vi "UTIL_RegEdit.vi"(9 "Mode":enum16{"Write", "Read", "Delete"}(ring), 10 "String Name":string="My String", 11 "String Value":string="LabVIEW") -> (2 "Success?":bool, 3 "Value Read":string)   [LabVIEW 2024]
doc: "This example demonstrates how to write, read, and delete a sample key from the Windows registry key HKEY_CURRENT_USER\\Allen_Aircraft\\. It will not affect the registry in any other way."
uses:
  <vilib>/registry/registry.llb/Registry RtKey.ctl
  <vilib>/registry/registry.llb/Write Registry Value Simple.vi
  <vilib>/registry/registry.llb/Read Registry Value Simple STR.vi
panel:
  # "Overview: Demonstrates the use of the Windows Registry Access VIs to write, read, and delete a sample key from the Windows registry.\nRequirements: Windows\nInstructions:\nRun the VI."
  # "KEY PATH:  HKEY_CURRENT_USER\\Allen_Aircraft\\Elevale_OLS_Test"
  # "See the diagram of this VI for more information on the Windows Registry Access VIs."
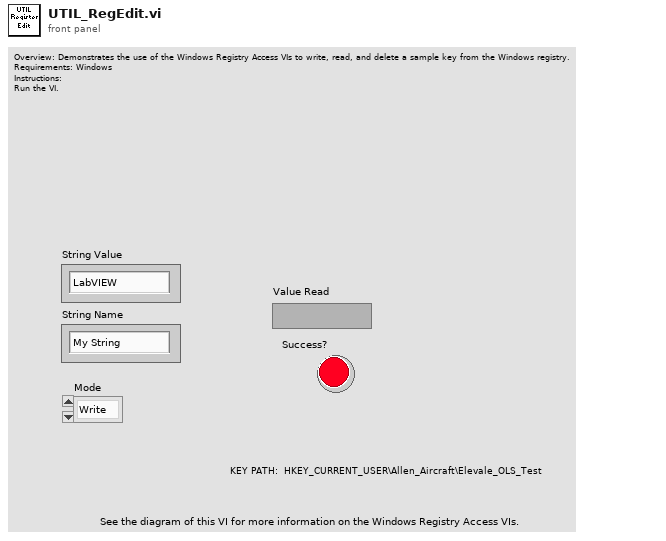
[diagram p1: front panel]
types:
  T1 = typedef "Registry RtKey.ctl" = enum32{"HKEY_CLASSES_ROOT", "HKEY_CURRENT_USER", "HKEY_LOCAL_MACHINE", "HKEY_USERS", "HKEY_PERFORMANCE_DATA", "HKEY_CURRENT_CONFIG", "HKEY_DYN_DATA"}
  T2 = typedef "Registry refnum.ctl" = refnum<k1>
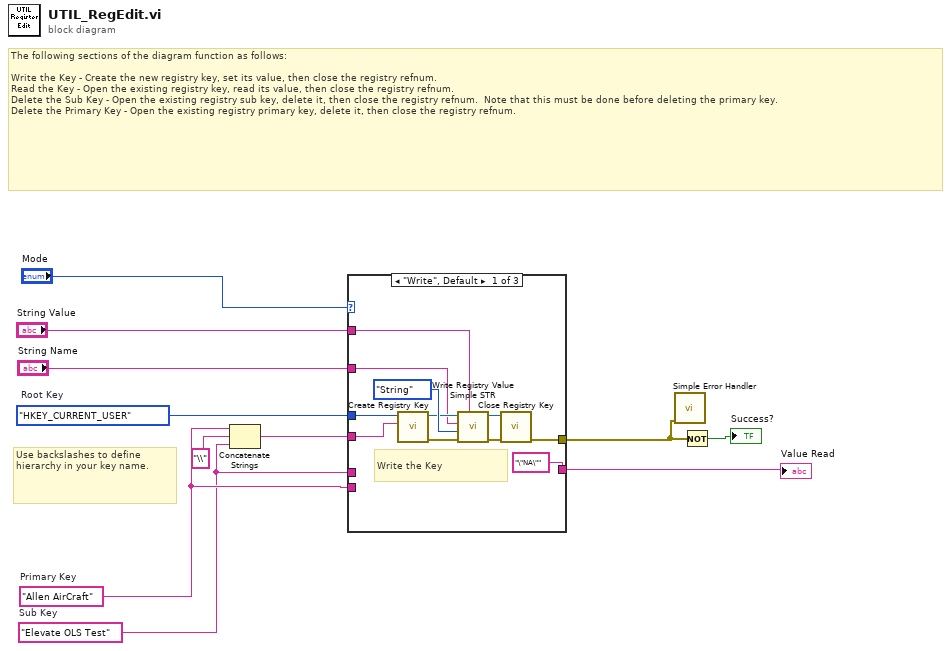
[diagram p0: block diagram]
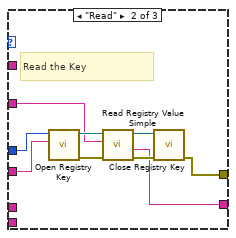
[diagram p2: hidden frame]
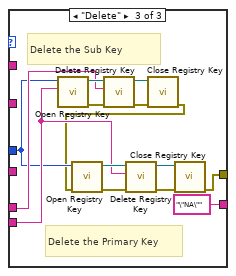
[diagram p3: hidden frame]
diagram:
  w2 = "Elevate OLS Test"  # Sub Key
  w3 = "Allen AirCraft"  # Primary Key
  w11 = Registry_RtKey."HKEY_CURRENT_USER"  # Root Key
  # "Use backslashes to define hierarchy in your key name."
  # "The following sections of the diagram function as follows:\n\nWrite the Key - Create the new registry key, set its value, then close the registry refnum.\nRead the Key - Open the existing registry key, read its value, then close the registry refnum.\nDelete the Sub Key - Open the existing registry sub key, delete it, then close the registry refnum.  Note that this must be done before deleting the primary key.\nDelete the Primary Key - Open the existing registry primary key, delete it, then close the registry refnum."
  n1 = Concatenate Strings(w3, "\\", w2) -> (w10:string)
  n2 = case shown="\"Write\", Default" "Mode" {
    tunnel: w11 -> [w17 w25 w35]
    tunnel: w10 -> [w16 w24 _]
    tunnel: [w15 w27 w33] -> w1
    tunnel: "String Name" -> [w14 w26 _]
    tunnel: "String Value" -> [w13 _ _]
    tunnel: ["\"NA\"" ("String/Binary data") w23 "\"NA\"" ("String/Binary data")] -> w4
    tunnel: w3 -> [_ _ w36]
    tunnel: w2 -> [_ _ w41]
    frame "Write", Default {
      # "Write the Key"
      n3 = call <vilib>:"Create Registry Key.vi"("subkey"=w16, "root key (HKEY_LOCAL_MACHINE)"=w17) -> ("error out"=w20:errorcluster, "refnum out"=w18:T2)  [unwired: 7 in, 1 out]
      n4 = call-poly <vilib>:"Write Registry Value Simple STR.vi"("String/Binary data"=w13, "error in (no error)"=w20, "simple data type"=enum16{"String", "Binary", "DWORD"}."String", "value"=w14, "refnum"=w18) -> ("error out"=w22:errorcluster, "refnum out"=w21:T2)  [unwired: 3 in]
      n5 = call <vilib>:"Close Registry Key.vi"("error in (no error)"=w22, "refnum"=w21) -> ("error out"=w15:errorcluster)  [unwired: 5 in]
    }
    frame "Read" {
      # "Read the Key"
      n6 = call <vilib>:"Open Registry Key.vi"("subkey"=w24, "root key (HKEY_LOCAL_MACHINE)"=w25) -> ("error out"=w31:errorcluster, "refnum out"=w30:T2)  [unwired: 8 in]
      n7 = call-poly <vilib>:"Read Registry Value Simple.vi"("error in (no error)"=w31, "value"=w26, "refnum"=w30) -> ("error out"=w28:errorcluster, "String/Binary data"=w23:string, "refnum out"=w29:T2)  [unwired: 3 in, 1 out]
      n8 = call <vilib>:"Close Registry Key.vi"("error in (no error)"=w28, "refnum"=w29) -> ("error out"=w27:errorcluster)  [unwired: 5 in]
    }
    frame "Delete" {
      # "Delete the Primary Key"
      # "Delete the Sub Key"
      n9 = call <vilib>:"Open Registry Key.vi"("subkey"=w36, "root key (HKEY_LOCAL_MACHINE)"=w35) -> ("error out"=w42:errorcluster, "refnum out"=w43:T2)  [unwired: 8 in]
      n10 = call <vilib>:"Delete Registry Key.vi"("error in (no error)"=w42, "subkey"=w41, "refnum"=w43) -> ("error out"=w44:errorcluster, "refnum out"=w45:T2)  [unwired: 7 in]
      n11 = call <vilib>:"Close Registry Key.vi"("error in (no error)"=w44, "refnum"=w45) -> ("error out"=w34:errorcluster)  [unwired: 5 in]
      n12 = call <vilib>:"Open Registry Key.vi"("error in (no error)"=w34, "root key (HKEY_LOCAL_MACHINE)"=w35) -> ("error out"=w38:errorcluster, "refnum out"=w37:T2)  [unwired: 8 in]
      n13 = call <vilib>:"Delete Registry Key.vi"("error in (no error)"=w38, "subkey"=w36, "refnum"=w37) -> ("error out"=w39:errorcluster, "refnum out"=w40:T2)  [unwired: 7 in]
      n14 = call <vilib>:"Close Registry Key.vi"("error in (no error)"=w39, "refnum"=w40) -> ("error out"=w33:errorcluster)  [unwired: 5 in]
    }
  }
  "Value Read" <- w4
  n15 = call <vilib>:"Simple Error Handler.vi"("error in (no error)"=w1) -> ()  [unwired: 4 in, 5 out]
  n16 = Not(x=w1) -> (.not. x?=→"Success?":bool)
